vi "Stop NMR Sweep.vi"   [LabVIEW 2010]
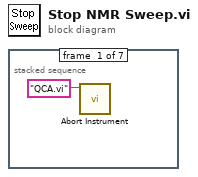
[diagram p0: block diagram]
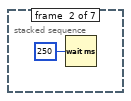
[diagram p2: hidden frame]
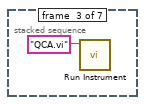
[diagram p3: hidden frame]
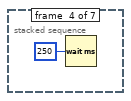
[diagram p4: hidden frame]
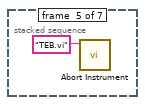
[diagram p5: hidden frame]
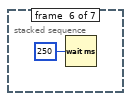
[diagram p6: hidden frame]
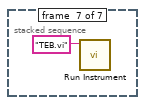
[diagram p7: hidden frame]
diagram:
  n1 = stacked-sequence {
    frame #0 {
      n2 = call <vilib>:"Abort Instrument.vi"("VI name"="QCA.vi") -> ()  [unwired: 10 in, 1 out]
    }
    frame #1 {
      n3 = Wait (ms)(milliseconds to wait=u32 250) -> ()  [unwired: 1 out]
    }
    frame #2 {
      n4 = call <vilib>:"Run Instrument.vi"("VI name"="QCA.vi") -> ()  [unwired: 10 in, 1 out]
    }
    frame #3 {
      n5 = Wait (ms)(milliseconds to wait=u32 250) -> ()  [unwired: 1 out]
    }
    frame #4 {
      n6 = call <vilib>:"Abort Instrument.vi"("VI name"="TEB.vi") -> ()  [unwired: 10 in, 1 out]
    }
    frame #5 {
      n7 = Wait (ms)(milliseconds to wait=u32 250) -> ()  [unwired: 1 out]
    }
    frame #6 {
      n8 = call <vilib>:"Run Instrument.vi"("VI name"="TEB.vi") -> ()  [unwired: 10 in, 1 out]
    }
  }
